vi "sensorPulso.vi"() -> ()   [LabVIEW 2014]
uses:
  FGV Machine states.ctl
  FGV Serial Folder/control/FGV Serial Tasks.ctl
panel:
  out "BPM":i32
  in  "threshold":i32
  out "Waveform Chart":i32(graph)
  in  "Haz clic en la carpeta:":path
  out "Status":u32(colorbox)
  in  "Pause":bool
  in  "Record":bool
  in  "exit":bool
  out "error out":errorcluster
  in  "Play Button":bool
  in  "stop":bool
  in  "Puerto serial":refnum<visa-resource-name>
  in  "error in (no error)":errorcluster
  in  "Cluster":T2={"Estado"=enum."Start", "Serial Port"="COM3", "Exit"=FALSE, "Timeout"=0, "filePath"=refnum, "isRecording"=FALSE, "valuesToTxt"="", "bpm"=0.0, "initialTime"=0.0, "actualTime"=0.0, "risingEdge"=FALSE, "fallingEdge"=FALSE}
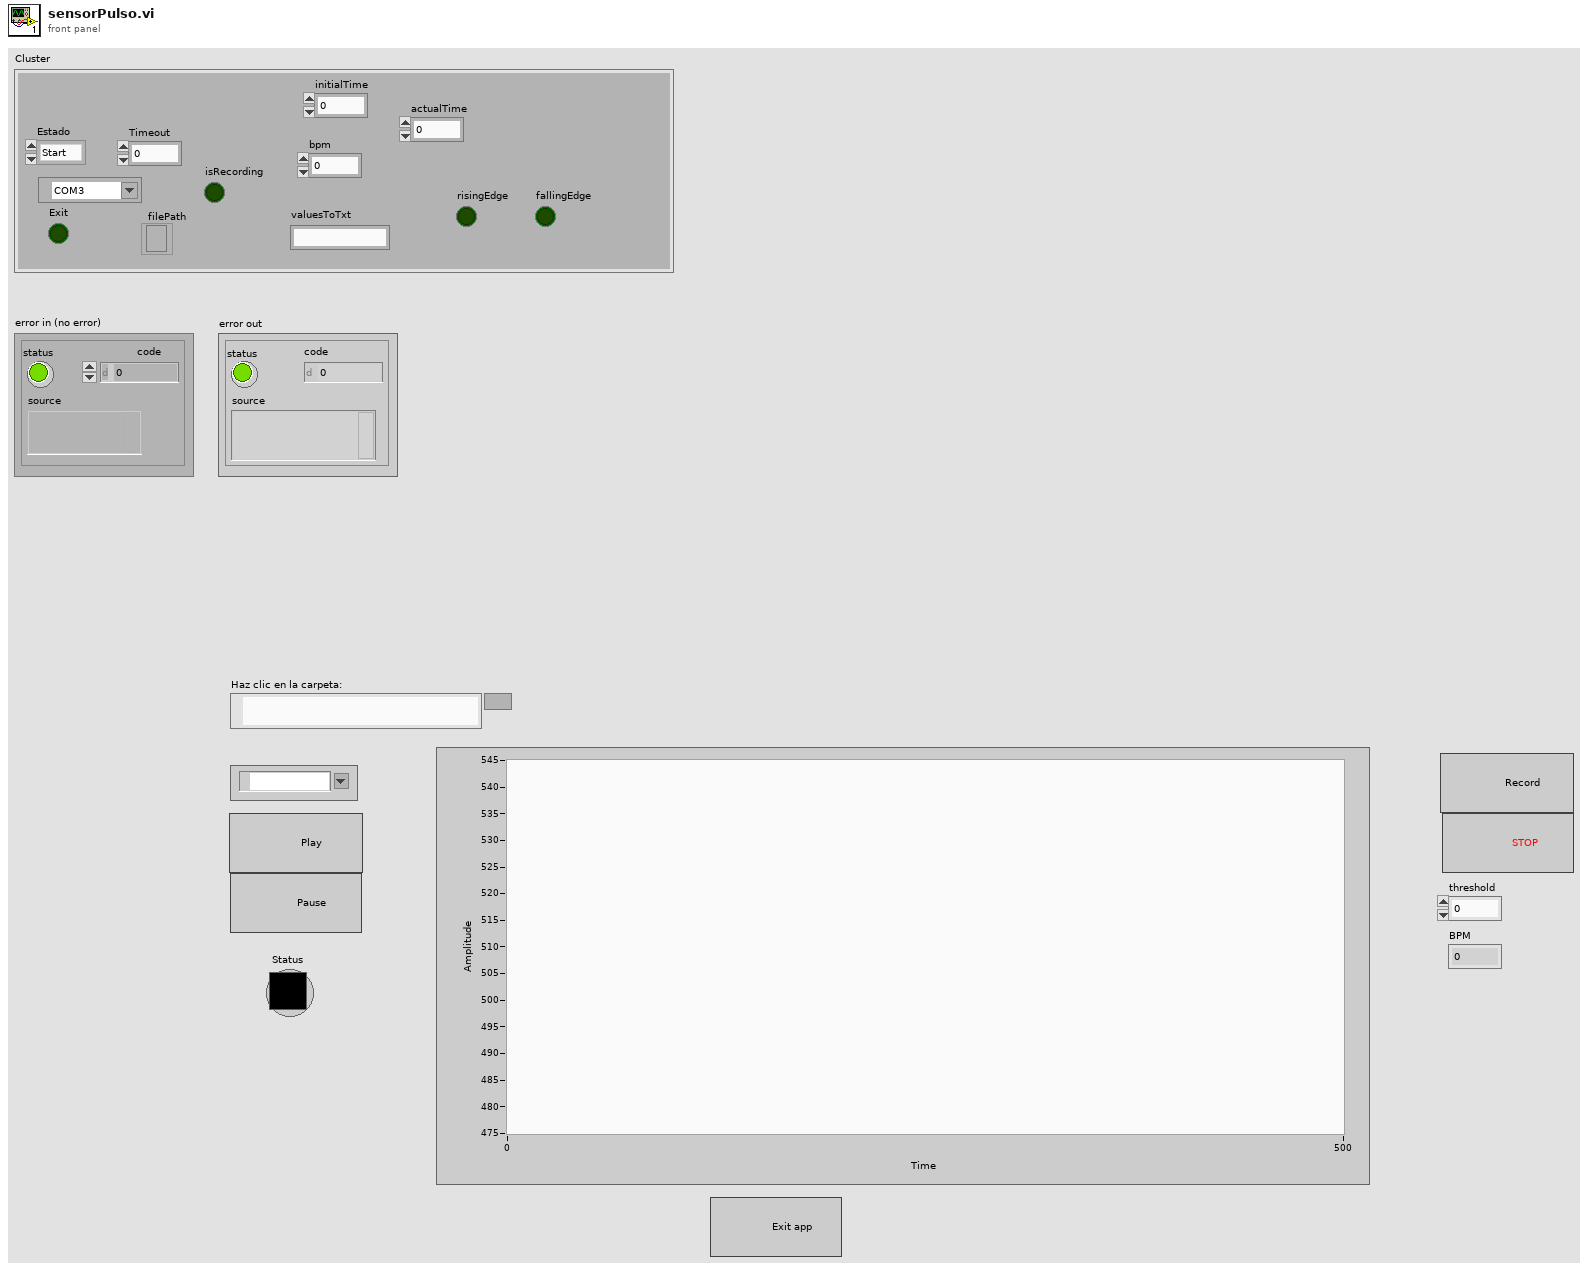
[diagram p1: front panel]
types:
  T1 = typedef "FGV Machine states.ctl" = enum16{"Init", "Start", "Wait", "Display", "Record", "Error handler", "Stop", "Pause", "Exit"}
  T2 = cluster{"Estado":T1, "Serial Port":refnum<visa-resource-name>, "Exit":bool, "Timeout":i32, "filePath":refnum<file>, "isRecording":bool, "valuesToTxt":string, "bpm":dbl, "initialTime":dbl, "actualTime":dbl, "risingEdge":bool, "fallingEdge":bool}
  T3 = typedef "FGV Serial Tasks.ctl" = enum16{"Open", "Read", "Write", "Close", "Flush"}
  T4 = enum16{"open", "replace", "create", "open or create", "replace or create", "replace or create with confirmation"}
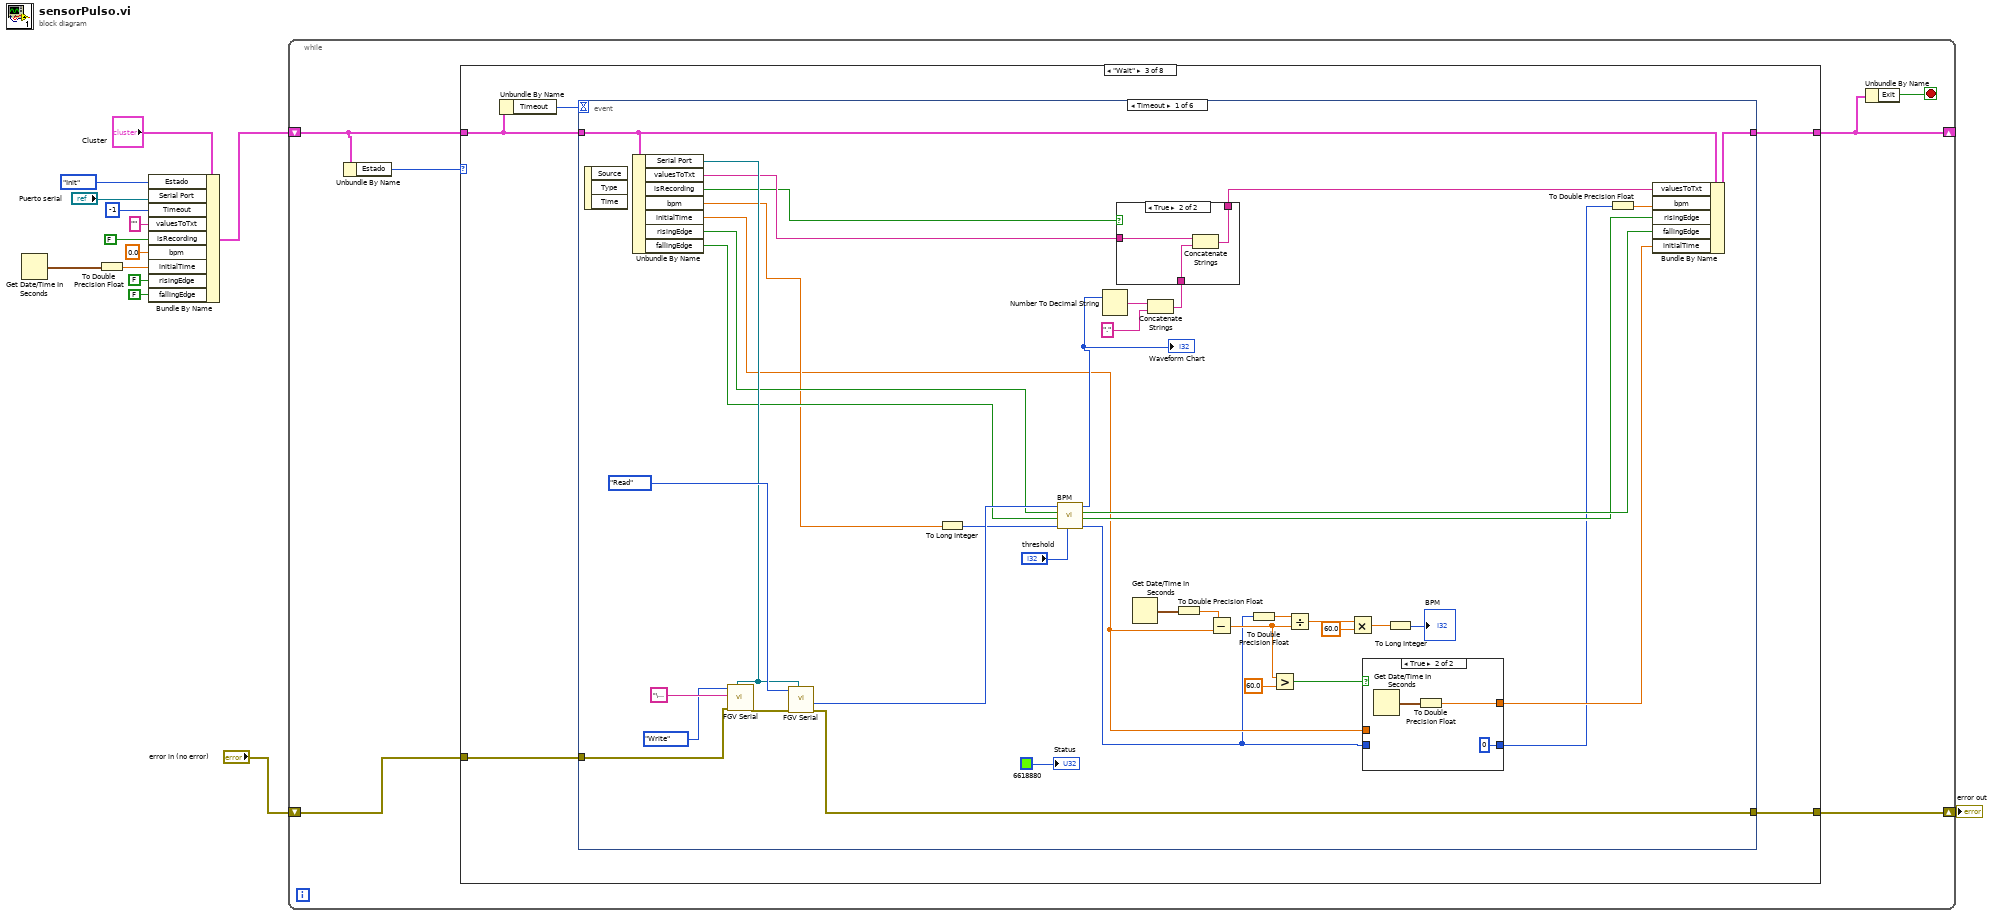
[diagram p0: block diagram]
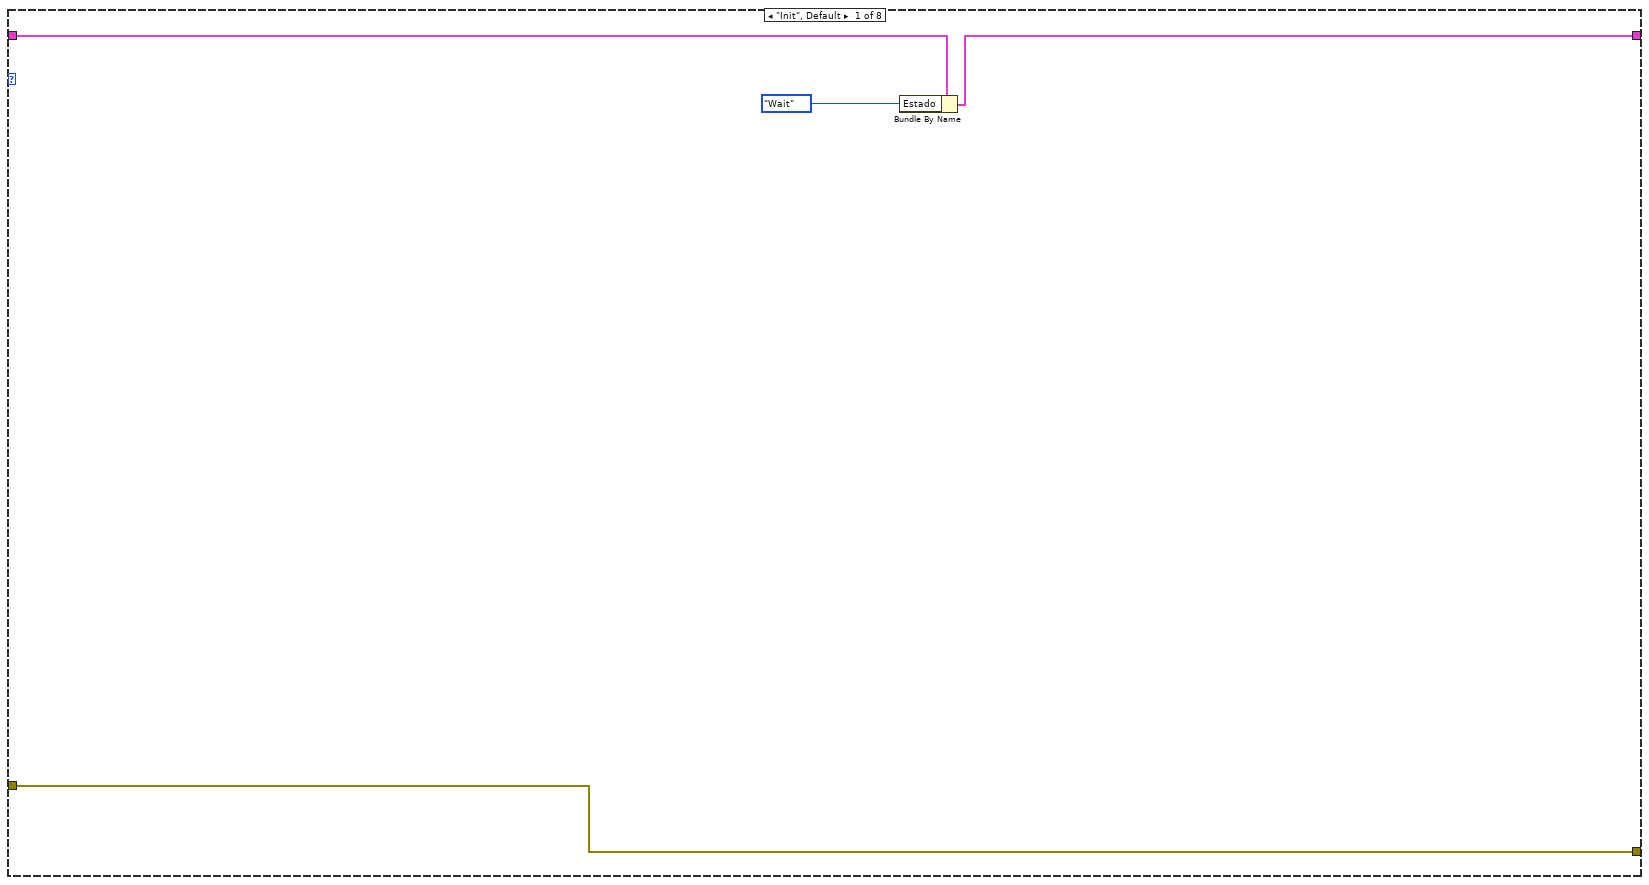
[diagram p2: hidden frame]
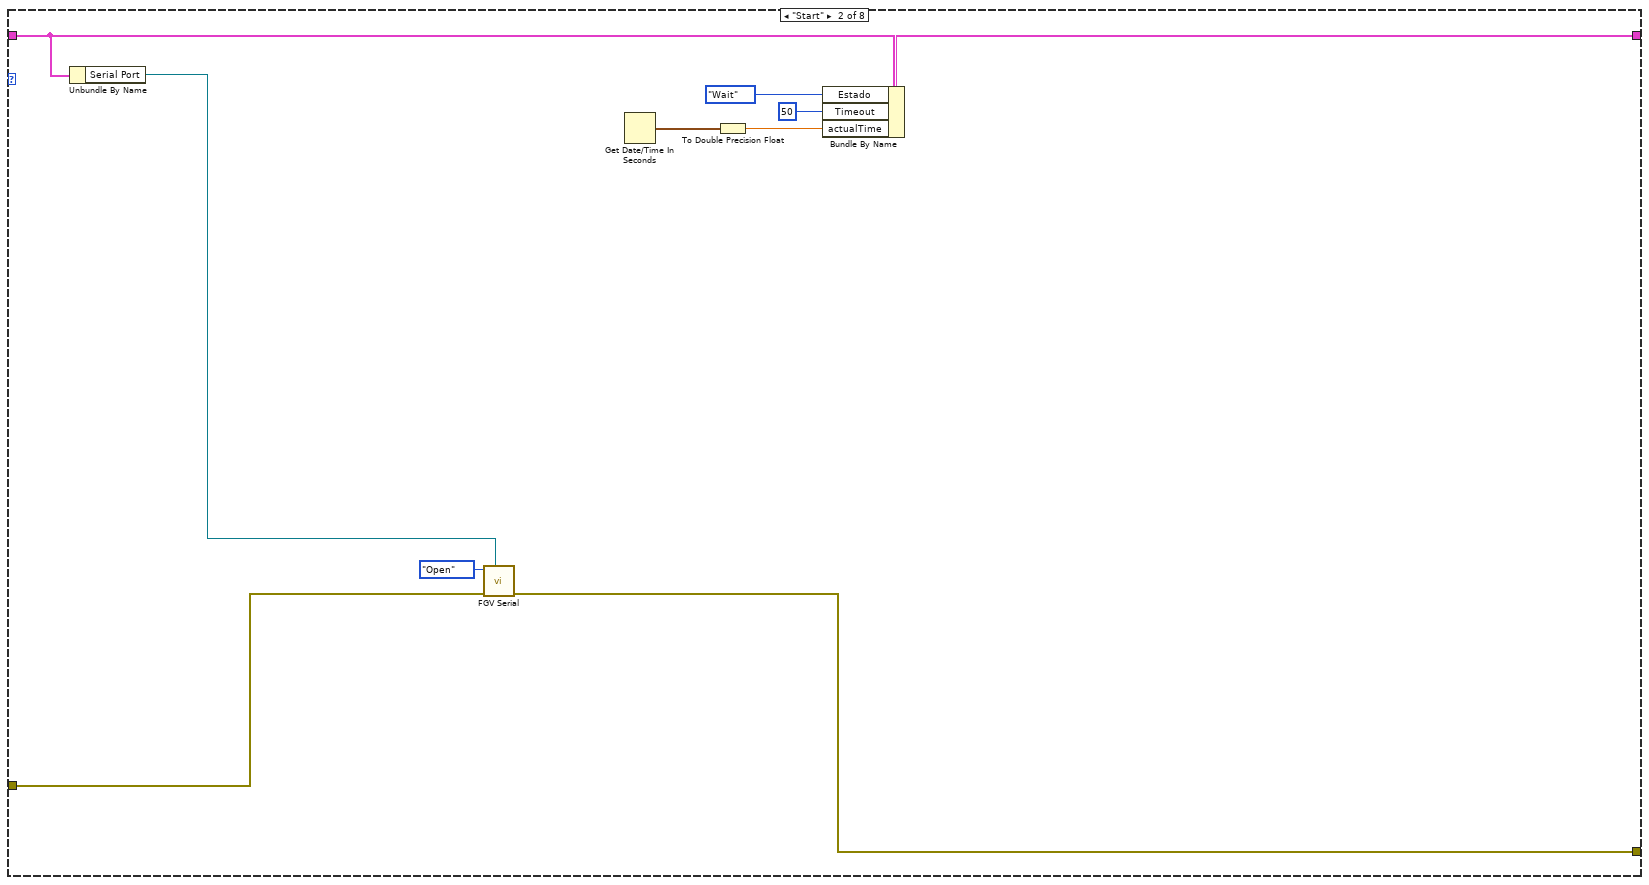
[diagram p3: hidden frame]
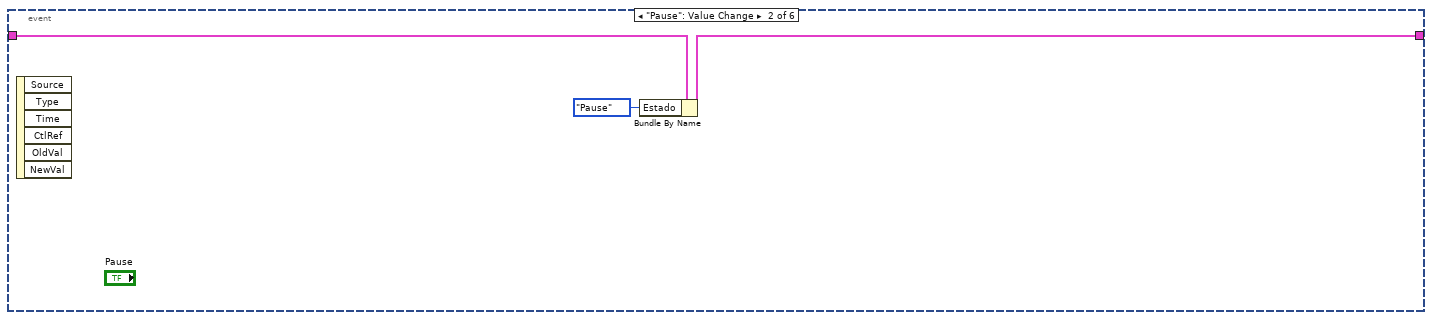
[diagram p6: hidden frame]
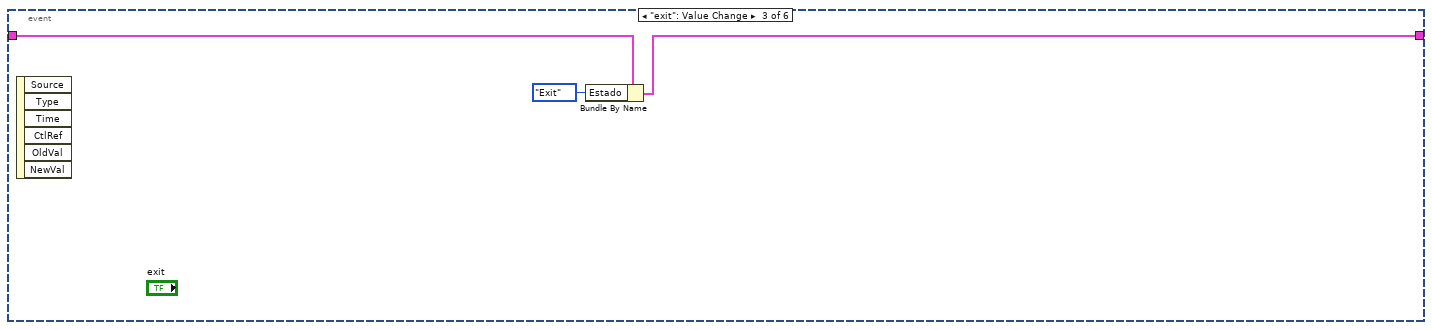
[diagram p7: hidden frame]
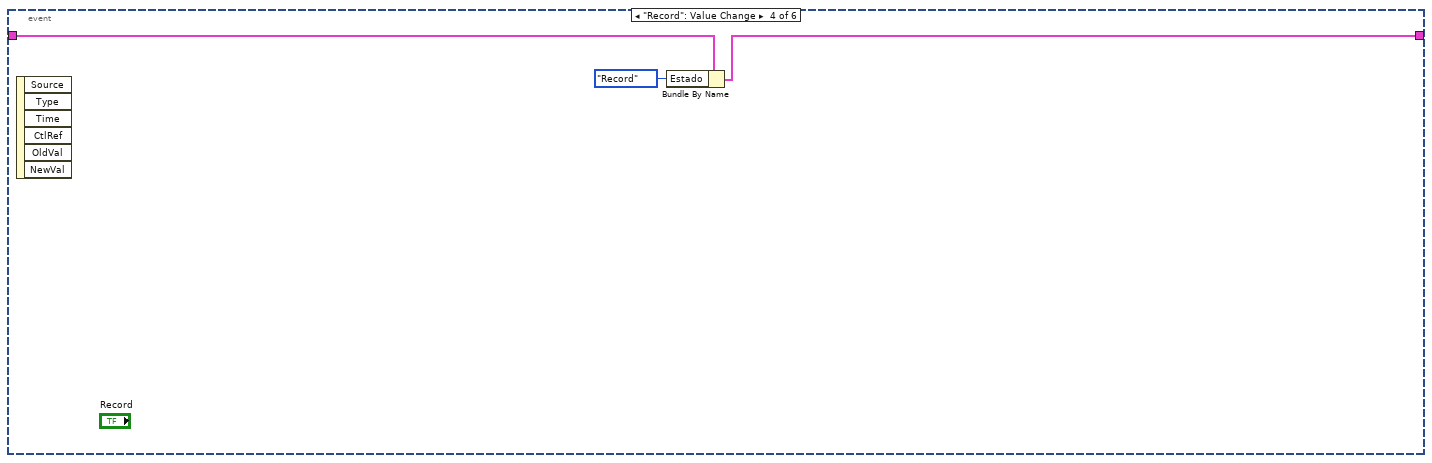
[diagram p8: hidden frame]
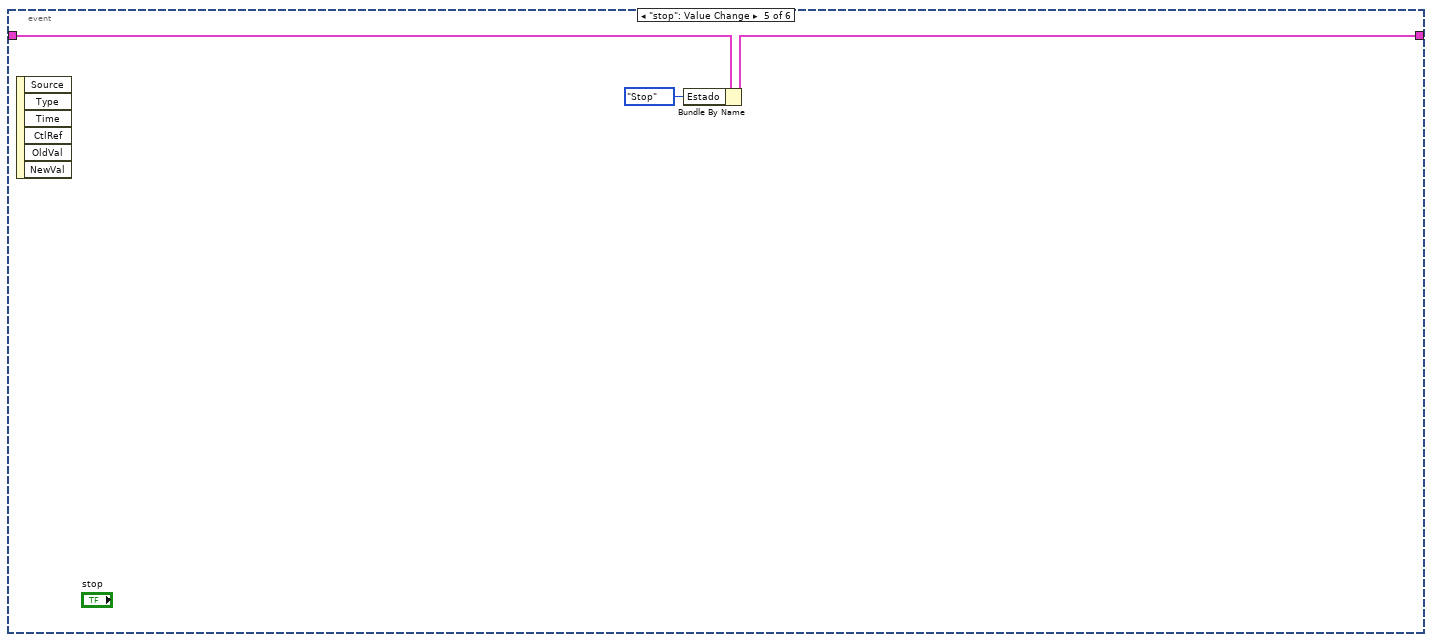
[diagram p9: hidden frame]
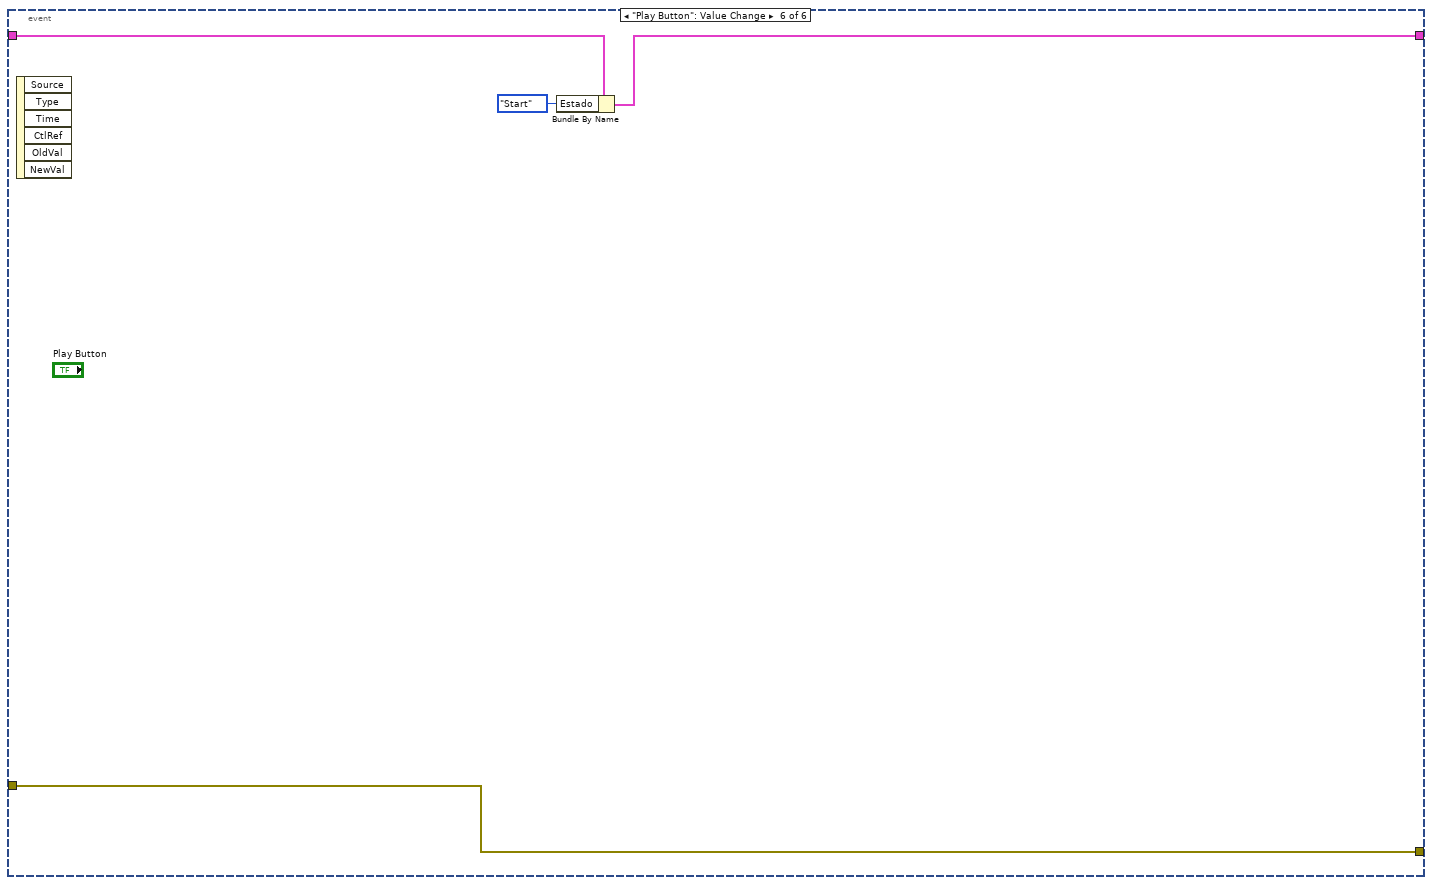
[diagram p10: hidden frame]
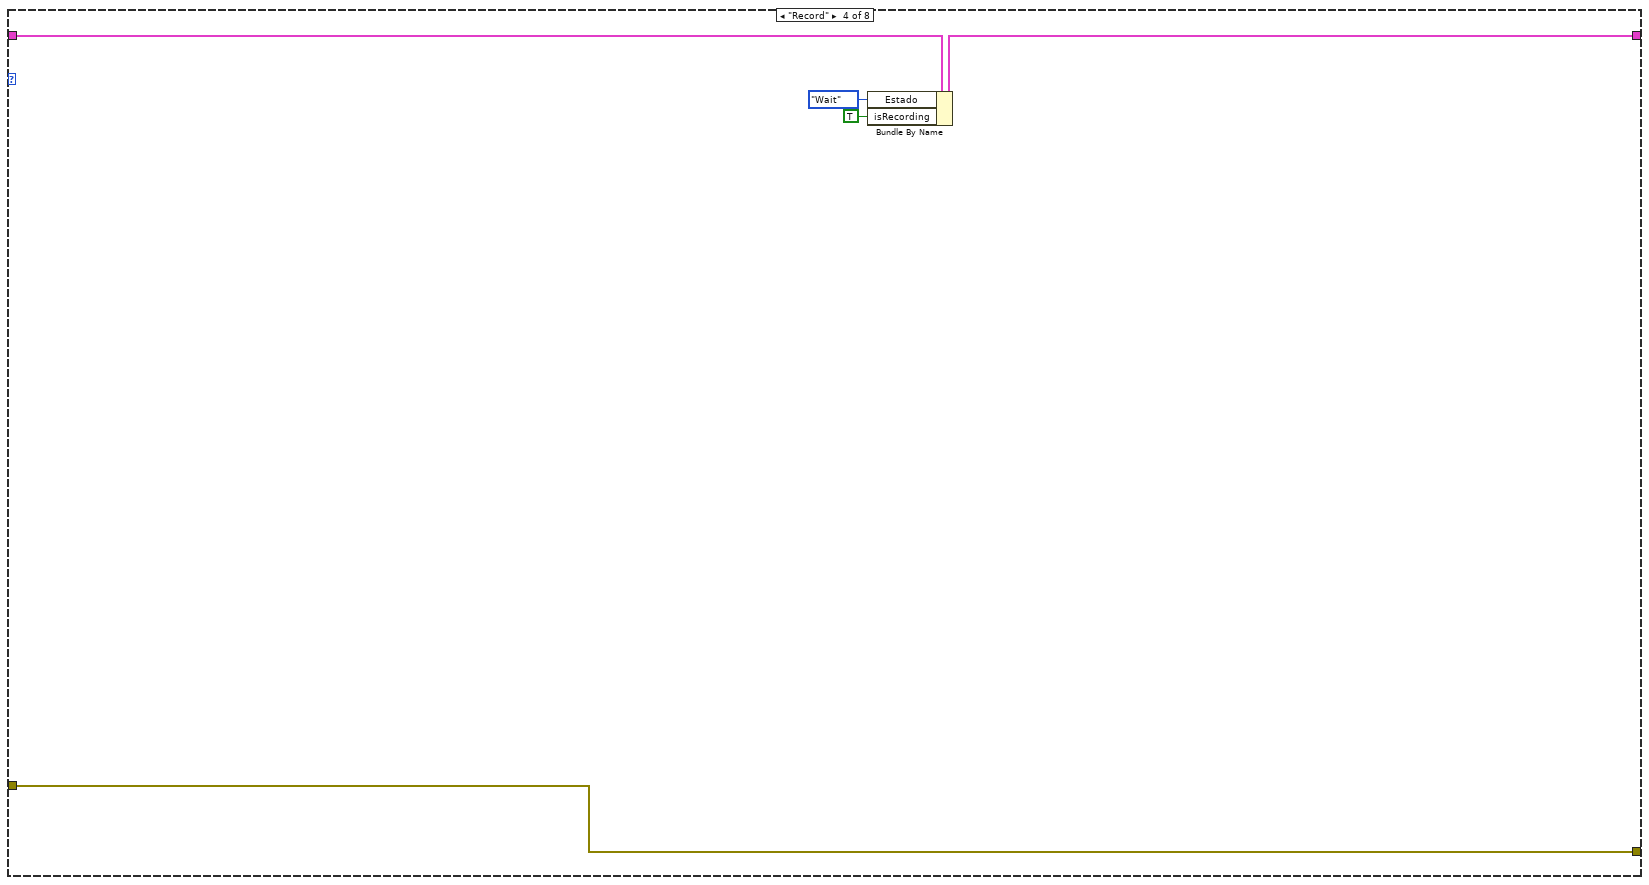
[diagram p11: hidden frame]
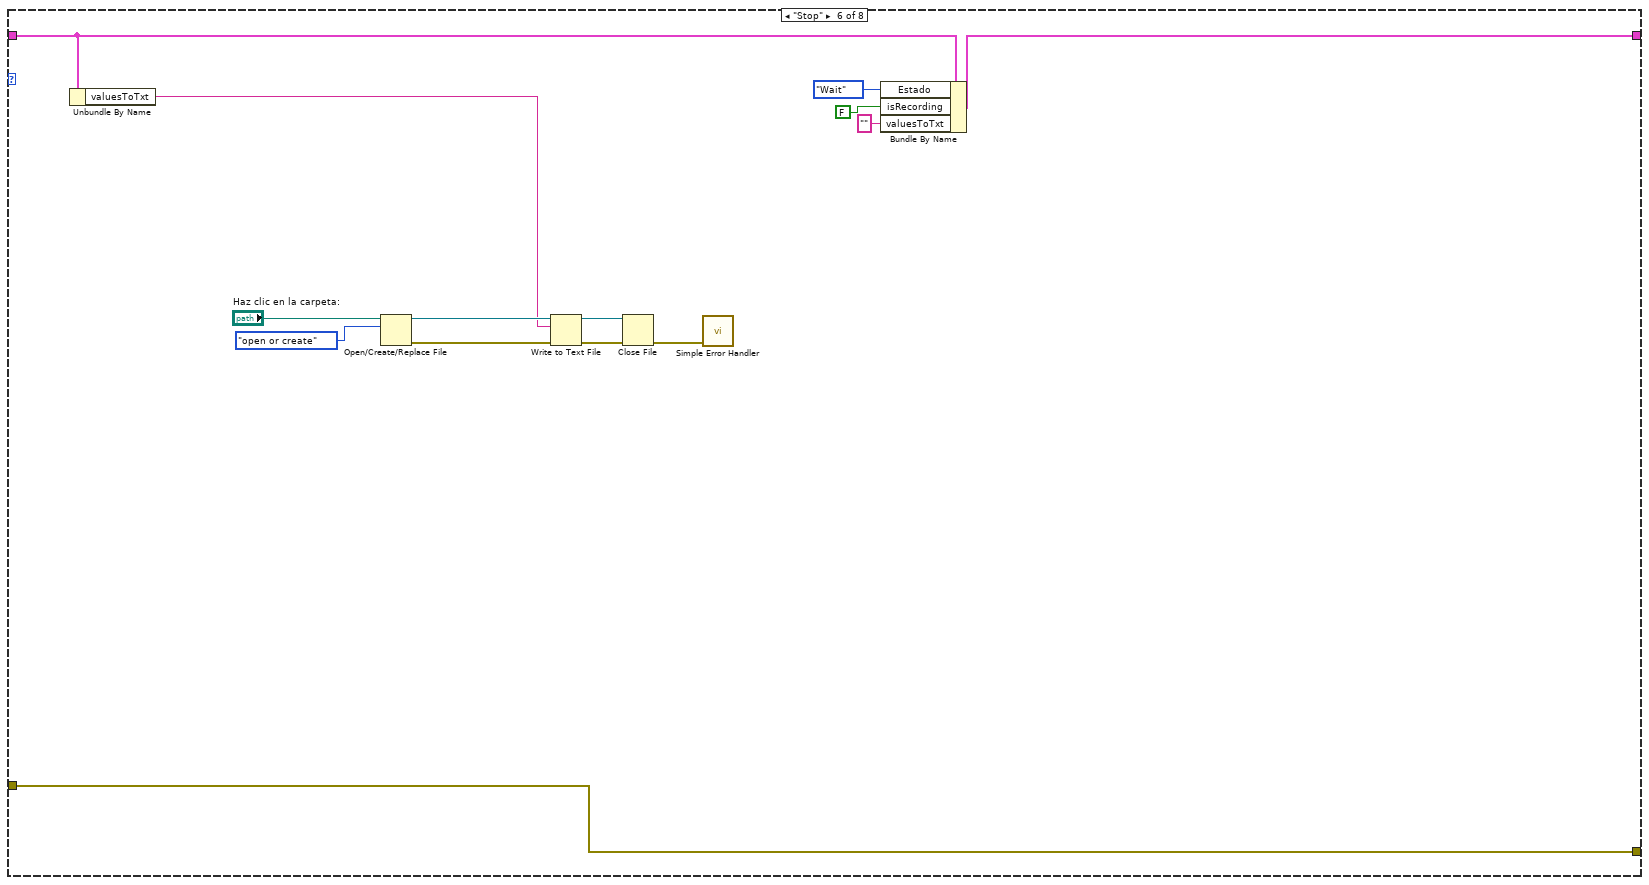
[diagram p13: hidden frame]
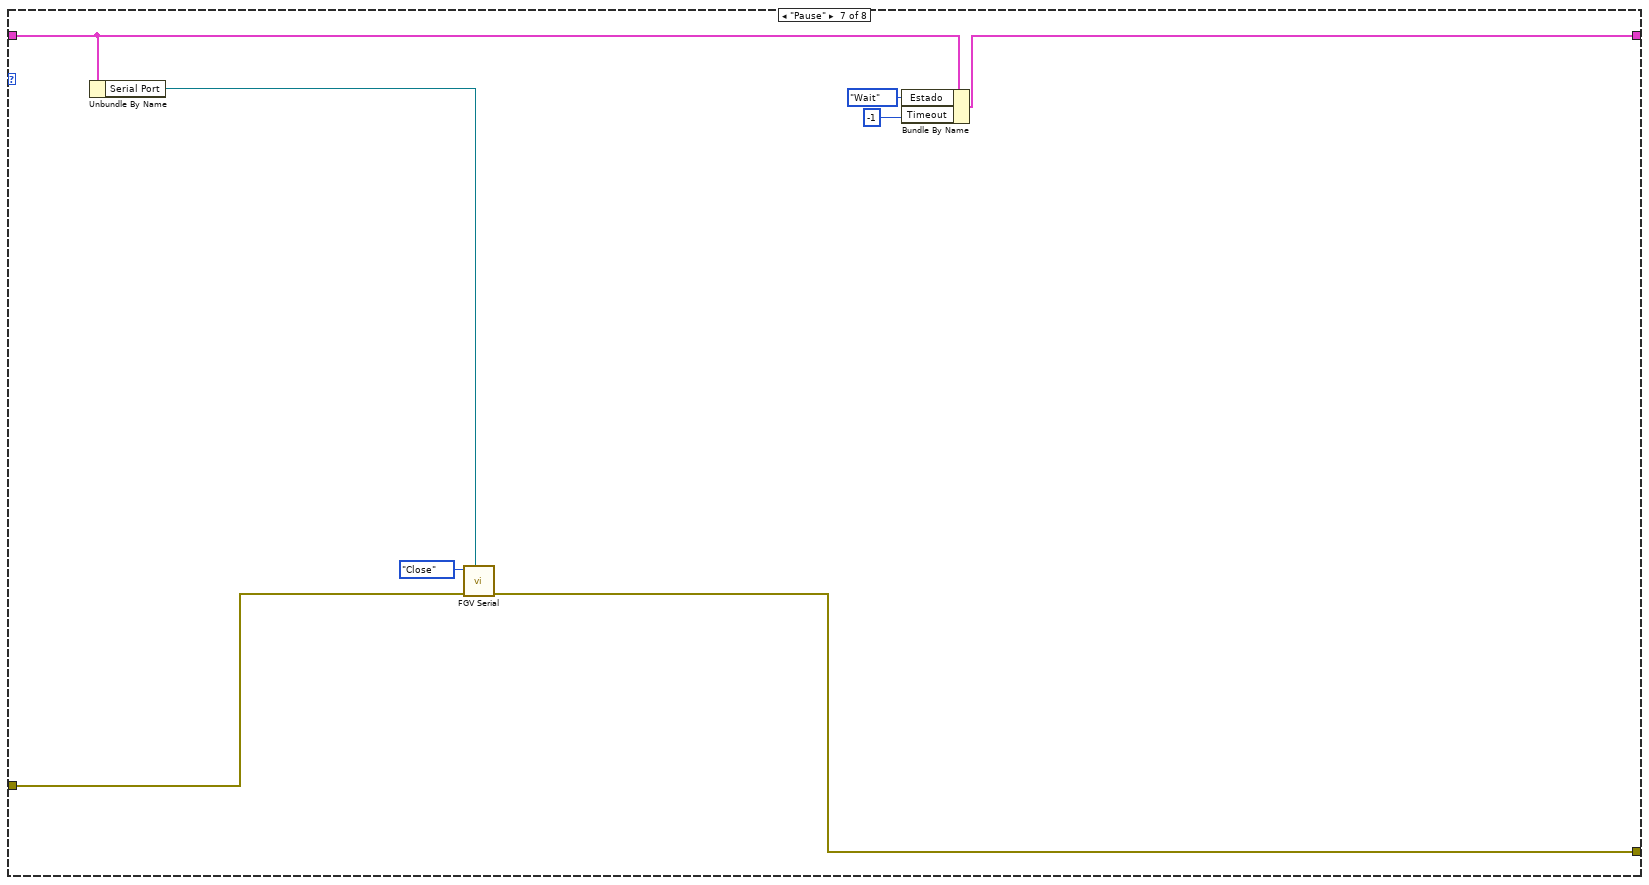
[diagram p14: hidden frame]
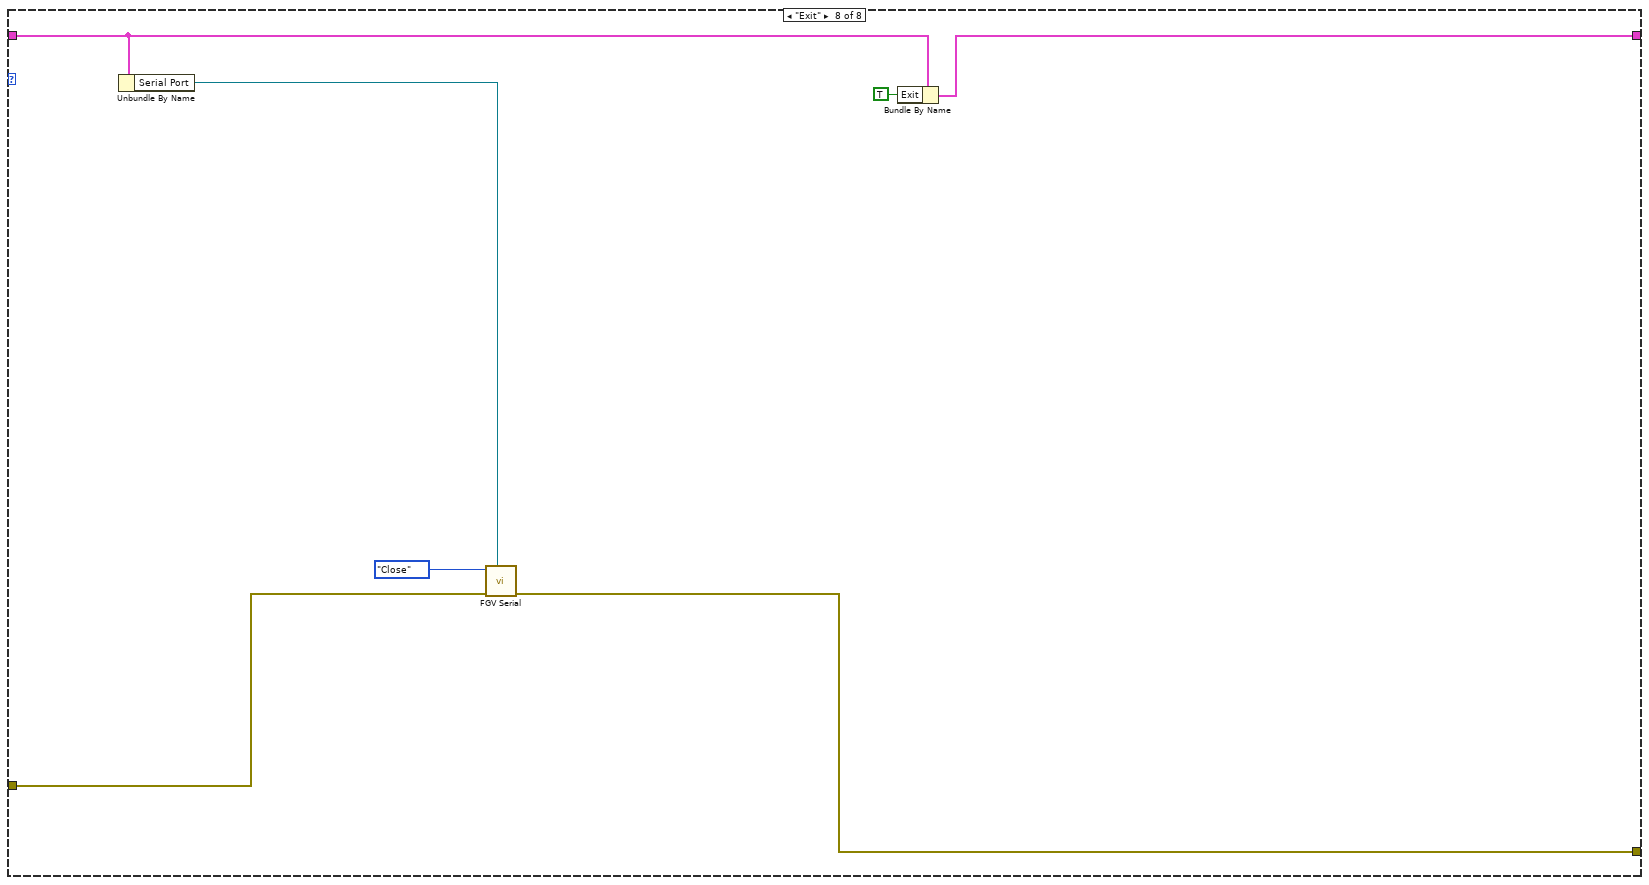
[diagram p15: hidden frame]
diagram:
  n1 = Get Date/Time In Seconds() -> (seconds since 1Jan1904=w3:timestamp)
  n2 = To Double Precision Float(number=w3) -> (double precision float=w4:dbl)
  n3 = Bundle By Name(cluster="Cluster", "Estado"=FGV_Machine_states."Init", "Serial Port"="Puerto serial", "Timeout"=-1, "valuesToTxt"="", "isRecording"=FALSE, "bpm"=0.0 ("filteredValue"), "initialTime"=w4, "risingEdge"=FALSE, "fallingEdge"=FALSE) -> (w10:T2)
  n4 = while {
    shift-right: [w15] -> _
    shift-left: w10 -> [w20]
    shift-right: [w17] -> w8
    shift-left: "error in (no error)" -> [w18]
    stop <- w16 stop-if-true
    n5 = Unbundle By Name(w20) -> ("Estado"=w19:T1)
    n6 = case shown="\"Wait\"" w19 {
      tunnel: [w23 w29 w39 w107 w111 w125 w128 w140] -> w15
      tunnel: w20 -> [w24 w30 w36 w108 w111 w121 w129 w136]
      tunnel: w18 -> [w21 w33 w38 w109 w110 w123 w132 w138]
      tunnel: [w21 w32 w37 w109 w110 w123 w131 w137] -> w17
      frame "Init", Default {
        n7 = Bundle By Name(cluster=w24, "Estado"=FGV_Machine_states."Wait") -> (w23:T2)
      }
      frame "Start" {
        n8 = Unbundle By Name(w30) -> ("Serial Port"=w31:refnum<visa-resource-name>)
        n9 = call "FGV Serial.vi"("VISA resource name"=w31, "error in (no error)"=w33, "Task"=FGV_Serial_Tasks."Open") -> ("error out"=w32:errorcluster)  [unwired: 6 in, 2 out]
        n10 = Get Date/Time In Seconds() -> (seconds since 1Jan1904=w26:timestamp)
        n11 = To Double Precision Float(number=w26) -> (double precision float=w25:dbl)
        n12 = Bundle By Name(cluster=w30, "Estado"=FGV_Machine_states."Wait", "Timeout"=50, "actualTime"=w25) -> (w29:T2)
      }
      frame "Wait" {
        n13 = Unbundle By Name(w36) -> ("Timeout"=w35:i32)
        n14 = event shown="[0] Timeout" {
          selector: _ -> [_ _ _ _ _ _]
          dyn-events: _ -> [_ _ _ _ _ _]
          timeout: w35 -> [_ _ _ _ _ _]
          tunnel: w36 -> [w69 w91 w94 w97 w100 w103]
          tunnel: [w68 w90 w93 w96 w99 w102] -> w39
          tunnel: w38 -> [w74 _ _ _ _ w104]
          tunnel: [w72 _ _ _ _ w104] -> w37
          event Timeout {
            n15 = event-data() -> ()  [unwired: 1 in, 3 out]
            n16 = Unbundle By Name(w69) -> ("Serial Port"=w76:refnum<visa-resource-name>, "valuesToTxt"=w71:string, "isRecording"=w67:bool, "bpm"=w59:dbl, "initialTime"=w43:dbl, "risingEdge"=w62:bool, "fallingEdge"=w61:bool)
            n17 = call "FGV Serial.vi"("VISA resource name"=w76, "error in (no error)"=w74, "String"="\u0001" ("write buffer"), "Task"=FGV_Serial_Tasks."Write") -> ("error out"=w75:errorcluster)  [unwired: 5 in, 2 out]
            n18 = call "FGV Serial.vi"("VISA resource name"=w76, "error in (no error)"=w75, "Task"=FGV_Serial_Tasks."Read") -> ("error out"=w72:errorcluster, "Text output"=w63:i32)  [unwired: 6 in, 1 out]
            n19 = To Long Integer(number=w59) -> (32bit integer=w60:i32)
            n20 = call "BPM.vi"("threshold"="threshold", "bpm"=w60, "fallingEdge"=w61, "risingEdge"=w62, "signal"=w63) -> ("outBPM"=w41:i32, "risingEdge_out"=w56:bool, "fallingEdge_out"=w57:bool, "outSignal"=w58:i32)  [unwired: 3 in]
            "Waveform Chart" <- w58
            n21 = Number To Decimal String(number=w58) -> (decimal integer string=w66:string)  [unwired: 1 in]
            n22 = Get Date/Time In Seconds() -> (seconds since 1Jan1904=w50:timestamp)
            n23 = Concatenate Strings(w66, "." ("string")) -> (w64:string)
            n24 = case shown="True" w67 {
              tunnel: w71 -> [w85 w88]
              tunnel: [w85 w87] -> w70
              tunnel: w64 -> [_ w86]
              frame False {
              }
              frame True {
                n25 = Concatenate Strings(w88, w86) -> (w87:string)
              }
            }
            n26 = To Double Precision Float(number=w50) -> (double precision float=w49:dbl)
            n27 = Subtract(x=w49, y=w43) -> (x-y=w46:dbl)
            n28 = To Double Precision Float(number=w41) -> (double precision float=w53:dbl)
            n29 = Greater?(x=w46, y=60.0) -> (0:w44:bool)
            n30 = Divide(x=w53, y=w46) -> (x/y=w52:dbl)
            n31 = Multiply(x=w52, y=60.0) -> (x*y=w48:dbl)
            n32 = case shown="True" w44 {
              tunnel: w43 -> [w81 _]
              tunnel: [w81 w83] -> w42
              tunnel: w41 -> [w80 _]
              tunnel: [w80 0 ("outBPM")] -> w40
              frame False {
              }
              frame True {
                n33 = Get Date/Time In Seconds() -> (seconds since 1Jan1904=w84:timestamp)
                n34 = To Double Precision Float(number=w84) -> (double precision float=w83:dbl)
              }
            }
            n35 = To Long Integer(number=w48) -> (32bit integer=→"BPM":i32)
            n36 = To Double Precision Float(number=w40) -> (double precision float=w55:dbl)
            n37 = Bundle By Name(cluster=w69, "valuesToTxt"=w70, "bpm"=w55, "risingEdge"=w56, "fallingEdge"=w57, "initialTime"=w42) -> (w68:T2)
            "Status" <- u32 6618880 ("Status")
          }
          event "Pause": Value Change {
            n38 = event-data() -> ()  [unwired: 1 in, 6 out]
            n39 = Bundle By Name(cluster=w91, "Estado"=FGV_Machine_states."Pause") -> (w90:T2)
          }
          event "exit": Value Change {
            n40 = event-data() -> ()  [unwired: 1 in, 6 out]
            n41 = Bundle By Name(cluster=w94, "Estado"=FGV_Machine_states."Exit") -> (w93:T2)
          }
          event "Record": Value Change {
            n42 = event-data() -> ()  [unwired: 1 in, 6 out]
            n43 = Bundle By Name(cluster=w97, "Estado"=FGV_Machine_states."Record") -> (w96:T2)
          }
          event "stop": Value Change {
            n44 = event-data() -> ()  [unwired: 1 in, 6 out]
            n45 = Bundle By Name(cluster=w100, "Estado"=FGV_Machine_states."Stop") -> (w99:T2)
          }
          event "Play Button": Value Change {
            n46 = event-data() -> ()  [unwired: 1 in, 6 out]
            n47 = Bundle By Name(cluster=w103, "Estado"=FGV_Machine_states."Start") -> (w102:T2)
          }
        }
      }
      frame "Record" {
        n48 = Bundle By Name(cluster=w108, "Estado"=FGV_Machine_states."Wait", "isRecording"=TRUE) -> (w107:T2)
      }
      frame "Error handler" {
      }
      frame "Stop" {
        n49 = Unbundle By Name(w121) -> ("valuesToTxt"=w112:string)
        n50 = Open/Create/Replace File(file path (use dialog)="Haz clic en la carpeta:", operation (0:open)=T4."open or create") -> (refnum out=w114:refnum<file>, error out=w113:errorcluster)  [unwired: 4 in, 1 out]
        n51 = Write to Text File(file (use dialog)=w114, text=w112, error in=w113) -> (refnum out=w119:refnum<file>, error out=w118:errorcluster)  [unwired: 1 in, 1 out]
        n52 = Close File(refnum=w119, error in=w118) -> (error out=w117:errorcluster)  [unwired: 1 out]
        n53 = call <vilib>:"Simple Error Handler.vi"("error in (no error)"=w117) -> ()  [unwired: 4 in, 5 out]
        n54 = Bundle By Name(cluster=w121, "Estado"=FGV_Machine_states."Wait", "isRecording"=FALSE, "valuesToTxt"="") -> (w125:T2)
      }
      frame "Pause" {
        n55 = Unbundle By Name(w129) -> ("Serial Port"=w130:refnum<visa-resource-name>)
        n56 = call "FGV Serial.vi"("VISA resource name"=w130, "error in (no error)"=w132, "Task"=FGV_Serial_Tasks."Close") -> ("error out"=w131:errorcluster)  [unwired: 6 in, 2 out]
        n57 = Bundle By Name(cluster=w129, "Estado"=FGV_Machine_states."Wait", "Timeout"=-1) -> (w128:T2)
      }
      frame "Exit" {
        n58 = Unbundle By Name(w136) -> ("Serial Port"=w135:refnum<visa-resource-name>)
        n59 = call "FGV Serial.vi"("VISA resource name"=w135, "error in (no error)"=w138, "Task"=FGV_Serial_Tasks."Close") -> ("error out"=w137:errorcluster)  [unwired: 6 in, 2 out]
        n60 = Bundle By Name(cluster=w136, "Exit"=TRUE) -> (w140:T2)
      }
    }
    n61 = Unbundle By Name(w15) -> ("Exit"=w16:bool)
  }
  "error out" <- w8
